vi "Post-Uninstall Custom Action.vi"(10 "Variant":variant) -> (0 "error out":errorcluster)   [LabVIEW 2017]
uses:
  <vilib>/Utility/sysdir.llb/System Directory Type.ctl
  <vilib>/xml/Load XML File.vi
  <vilib>/xml/NI_XML.lvlib
  <resource>/objmgr/DOMUserDefRef.rc
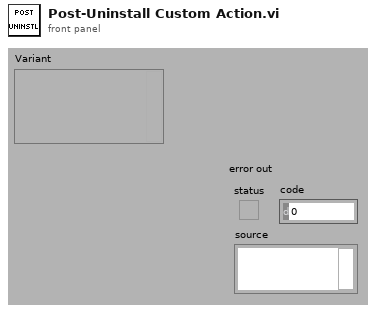
[diagram p1: front panel]
types:
  T1 = typedef "System Directory Type.ctl" = i32
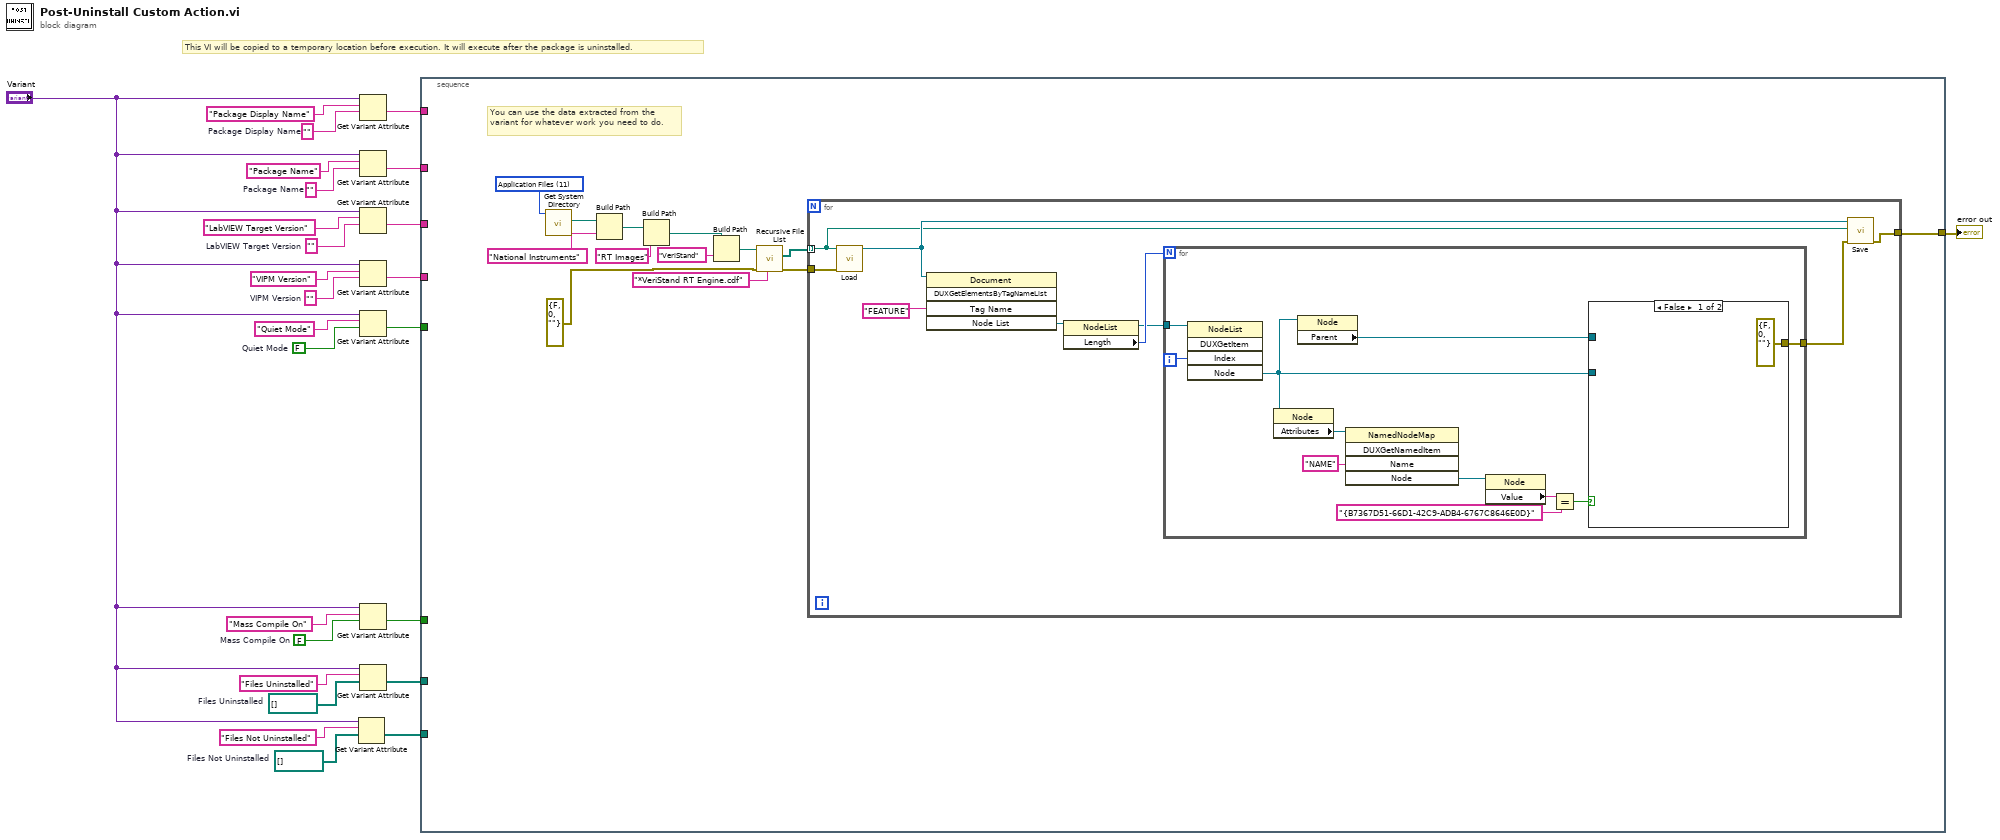
[diagram p0: block diagram]
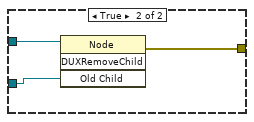
[diagram p2: hidden frame]
diagram:
  w2 = path[] []  # Files Not Uninstalled
  w3 = path[] []  # Files Uninstalled
  w9 = FALSE  # Mass Compile On
  w10 = ""  # Package Display Name
  w17 = FALSE  # Quiet Mode
  w20 = ""  # VIPM Version
  w22 = ""  # LabVIEW Target Version
  w24 = ""  # Package Name
  # "This VI will be copied to a temporary location before execution. It will execute after the package is uninstalled."
  n1 = Get Variant Attribute(Variant="Variant", name="Files Not Uninstalled", default value (empty Variant)=w2) -> (value=w7:path[])  [unwired: 1 in, 3 out]
  n2 = Get Variant Attribute(Variant="Variant", name="Package Display Name", default value (empty Variant)=w10) -> (value=w16:string)  [unwired: 1 in, 3 out]
  n3 = Get Variant Attribute(Variant="Variant", name="Package Name", default value (empty Variant)=w24) -> (value=w15:string)  [unwired: 1 in, 3 out]
  n4 = Get Variant Attribute(Variant="Variant", name="LabVIEW Target Version", default value (empty Variant)=w22) -> (value=w14:string)  [unwired: 1 in, 3 out]
  n5 = Get Variant Attribute(Variant="Variant", name="VIPM Version", default value (empty Variant)=w20) -> (value=w13:string)  [unwired: 1 in, 3 out]
  n6 = Get Variant Attribute(Variant="Variant", name="Quiet Mode", default value (empty Variant)=w17) -> (value=w12:bool)  [unwired: 1 in, 3 out]
  n7 = Get Variant Attribute(Variant="Variant", name="Mass Compile On", default value (empty Variant)=w9) -> (value=w11:bool)  [unwired: 1 in, 3 out]
  n8 = Get Variant Attribute(Variant="Variant", name="Files Uninstalled", default value (empty Variant)=w3) -> (value=w6:path[])  [unwired: 1 in, 3 out]
  n9 = stacked-sequence {
    tunnel: w16 -> [_]
    tunnel: w15 -> [_]
    tunnel: w14 -> [_]
    tunnel: w13 -> [_]
    tunnel: w12 -> [_]
    tunnel: w11 -> [_]
    tunnel: w6 -> [_]
    tunnel: w7 -> [_]
    tunnel: [w28] -> w1
    frame #0 {
      w31 = T1 11 items=["User Home"=0, "User Desktop"=1, "User Documents"=2, "User Application Data"=3, "User Preferences"=4, "User Temporary"=5, "Public Documents"=6, "Public Application Data"=7, "Public Preferences"=8, "Public Cache"=13, "System Core Libraries"=9, "System Installed Libraries"=10, "Application Files"=11, "Boot Volume Root"=12] ("system directory type")
      # "You can use the data extracted from the variant for whatever work you need to do."
      n10 = call <vilib>:"Get System Directory.vi"("system directory type"=w31) -> ("system directory"=w39:path)  [unwired: 10 in]
      n11 = Build Path(base path=w39, name or relative path="National Instruments") -> (appended path=w37:path)
      n12 = Build Path(base path=w37, name or relative path="RT Images") -> (appended path=w32:path)
      n13 = Build Path(base path=w32, name or relative path="VeriStand") -> (appended path=w34:path)
      n14 = call <vilib>:"Recursive File List.vi"("pattern"="*VeriStand RT Engine.cdf", "error in (no error)"=errorcluster {"status"=FALSE, "code"=0, "source"=""} ("error out"), "Folder Path"=w34) -> ("error out"=w29:errorcluster, "All Files in Dir"=w27:path[])  [unwired: 4 in, 3 out]
      n15 = for {
        tunnel: w27 -> [w40] mode=indexing
        tunnel: w29 -> [w48]
        tunnel: [w41] -> w28
        n16 = call-poly <vilib>:"Load.vi"("path to XML document"=w40, "error in (no error)"=w48) -> ("DOM document out"=w43:refnum<k20>)  [unwired: 11 in, 2 out]
        n17 = invoke class="Document" method="DUXGetElementsByTagNameList"(reference=w43, "Tag Name"="FEATURE") -> ("Node List"=w46:refnum<k20>)  [unwired: 3 in, 4 out]
        n18 = property class="NodeList"(reference=w46) -> (reference out=w44:refnum<k20>, "Length"=w45:i32)  [unwired: 1 in, 1 out]
        n19 = for {
          N: w45 -> [_]
          tunnel: w44 -> [w59]
          tunnel: [w49] -> w42
          i -> [w58]
          n20 = invoke class="NodeList" method="DUXGetItem"(reference=w59, "Index"=w58) -> ("Node"=w51:refnum<k20>)  [unwired: 3 in, 4 out]
          n21 = property class="Node"(reference=w51) -> ("Attributes"=w57:refnum<k20>)  [unwired: 1 in, 2 out]
          n22 = property class="Node"(reference=w51) -> ("Parent"=w50:refnum<k20>)  [unwired: 1 in, 2 out]
          n23 = invoke class="NamedNodeMap" method="DUXGetNamedItem"(reference=w57, "Name"="NAME") -> ("Node"=w55:refnum<k20>)  [unwired: 3 in, 4 out]
          n24 = property class="Node"(reference=w55) -> ("Value"=w54:string)  [unwired: 1 in, 2 out]
          n25 = Equal?(x=w54, y="{B7367D51-66D1-42C9-ADB4-6767C8646E0D}") -> (x = y?=w52:bool)
          n26 = case shown="False" w52 {
            tunnel: w51 -> [_ w62]
            tunnel: w50 -> [_ w63]
            tunnel: [errorcluster {"status"=FALSE, "code"=0, "source"=""} ("error out") w61] -> w49
            frame False {
            }
            frame True {
              n27 = invoke class="Node" method="DUXRemoveChild"(reference=w63, "Old Child"=w62) -> (error out=w61:errorcluster)  [unwired: 2 in, 3 out]
            }
          }
        }
        n28 = call <vilib>:"Save.vi"("error in (no error)"=w42, "XML file path"=w40, "DOM document in"=w43) -> ("error out"=w41:errorcluster)  [unwired: 6 in, 2 out]
      }
    }
  }
  "error out" <- w1
